vi "epsilon global.vi"() -> ()   [LabVIEW 2014, in "NI_AALPro.lvlib"]
uses:
  NI_AALPro.lvlib
panel:
  in  "eps for remove zeros":dbl=2.220446049250313e-16
  in  "eps for GCD":dbl=1e-10
  in  "eps for nth div of p/q":dbl=1e-10
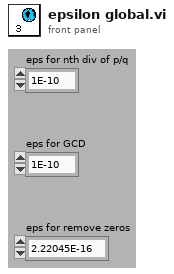
[diagram p1: front panel]
diagram:
